vi "APC_AppendUnits.vi"(1 "units":string[](array[string]), 2 "names":string[](array[string])) -> (0 "names_units":string[](array[string]))   [LabVIEW 2020]
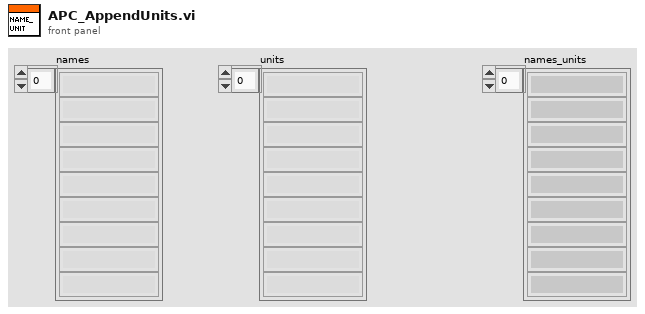
[diagram p1: front panel]
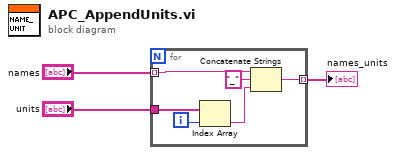
[diagram p0: block diagram]
diagram:
  n1 = for {
    tunnel: "names" -> [w9] mode=indexing
    tunnel: "units" -> [w6]
    tunnel: [w7] -> w2 mode=indexing
    i -> [w4]
    n2 = Index Array(array=w6, index=w4) -> (element=w5:string)
    n3 = Concatenate Strings(w9, "_" ("string"), w5) -> (w7:string)
  }
  "names_units" <- w2
